vi "Write Bytestreams to stdin.vi"(10 "data":refnum<class "Bytestream.lvclass">[](array[class]), 11 "subprocess in":refnum<class "Buffered Subprocess.lvclass">) -> (3 "subprocess out":refnum<class "Buffered Subprocess.lvclass">)   [LabVIEW 2020, in "NI_Subprocess.lvlib" / "Buffered Subprocess.lvclass"]
uses:
  <vilib>/Subprocess/Buffered Subprocess/Buffered Subprocess.lvclass
  <vilib>/Array/Bytestream/Bytestream.lvclass
  <vilib>/Subprocess/Buffered Subprocess/Buffered Subprocess.lvclass/Buffered Subprocess.ctl
  445baf28-d834-3fc7-00d5-7d1d1cfccc3f.vi
  <vilib>/Array/Bytestream/Concatenate Array.vi
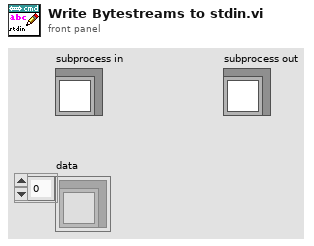
[diagram p1: front panel]
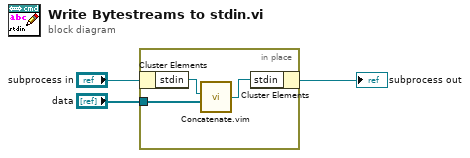
[diagram p0: block diagram]
diagram:
  n1 = in-place {
    in-place-border: "data" -> [w4]
    n2 = in-place-cluster #1("subprocess in") -> ("stdin"=w6:refnum<class "Bytestream.lvclass">)
    n3 = call "Concatenate.vim"("b"=w4, "a"=w6) -> ("a+b"=w5:refnum<class "Bytestream.lvclass">)  [unwired: 2 in]
    n4 = in-place-cluster #1("stdin"=w5) -> (→"subprocess out":refnum<class "Buffered Subprocess.lvclass">)
  }
